vi "triggerMechanism.vi"() -> ()   [LabVIEW 2017]
uses:
  <vilib>/eio/EIONode/EIONode.xnode
  <vilib>/rvi/eio/common/nirviEmuTemplateMethod_errors.vi
panel:
  out "Connector2/DIO26":bool
  out "Numeric":i16
  out "x .xor. y?":bool
  in  "Connector2/DIO12":bool
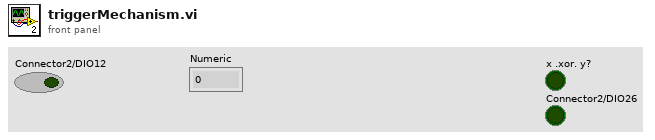
[diagram p1: front panel]
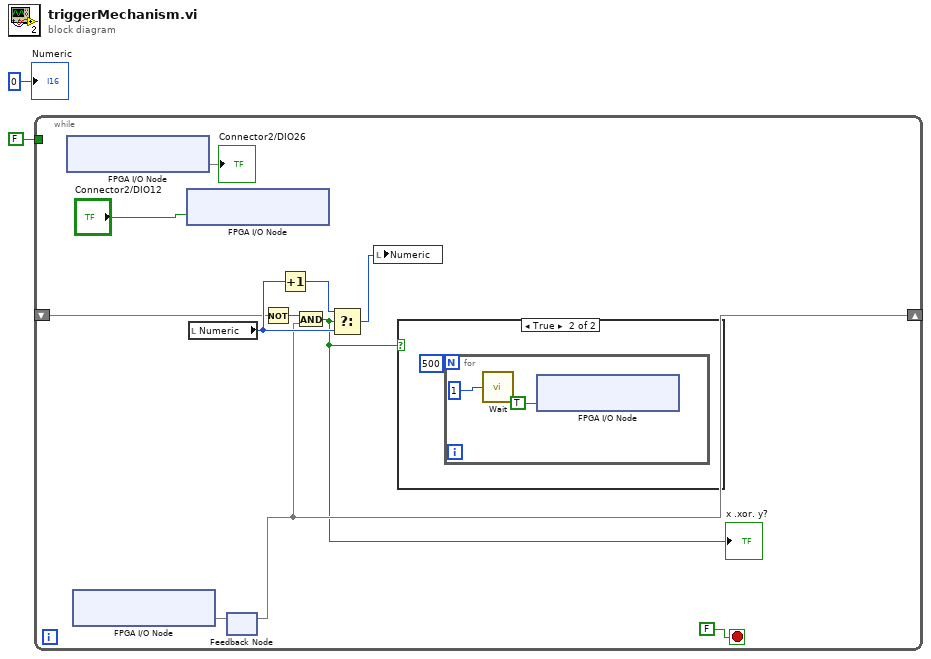
[diagram p0: block diagram]
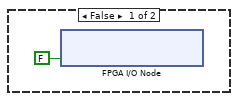
[diagram p2: hidden frame]
diagram:
  n1 = while {
    tunnel: FALSE ("initialize") -> [_]
    shift-right: [w4] -> _
    shift-left: _ -> [w5]
    stop <- FALSE stop-if-true
    n2 = xnode "FPGA I/O Node"() -> ("Connector2/DIO26"=→"Connector2/DIO26")  [unwired: 1 in, 1 out]
    n3 = xnode "FPGA I/O Node"() -> ("Connector2/DIO12"=w12)  [unwired: 1 in, 1 out]
    n4 = xnode "FPGA I/O Node"("Connector2/DIO12"="Connector2/DIO12") -> ()  [unwired: 1 in, 1 out]
    n5 = local read "Numeric"() -> (w8:i16)
    n6 = feedback-in #1(w12) -> ()
    n7 = feedback #1() -> (w4)  [unwired: 1 in]
    n8 = Not(x=w5) -> (.not. x?=w6:bool)
    n9 = Increment(x=w8) -> (x+1=w10:i16)
    n10 = And(x=w6, y=w4) -> (x .and. y?=w3:bool)
    "x .xor. y?" <- w3
    n11 = Select(t=w10, s=w3, f=w8) -> (s? t:f=w9:i16)
    n12 = local write "Numeric"(w9) -> ()
    n13 = case shown="True" w3 {
      frame False {
        n14 = xnode "FPGA I/O Node"("Connector2/DIO26"=FALSE) -> ()  [unwired: 1 in, 1 out]
      }
      frame True {
        n15 = for {
          N: 500 -> [_]
          n16 = call "Wait"("Count(uSec)"=u32 1) -> ()  [unwired: 1 out]
          n17 = xnode "FPGA I/O Node"("Connector2/DIO26"=TRUE) -> ()  [unwired: 1 in, 1 out]
        }
      }
    }
  }
  "Numeric" <- i16 0 ("Numeric")
